vi "Checkers Main Menu.vi"() -> ()   [LabVIEW 2016]
uses:
  Game Info Global Variable.vi
panel:
  in  "SETTINGS":bool
  in  "HOW TO PLAY":bool
  in  "Comp Name:":string="Computer"
  in  "LOAD SAVED GAME":bool
  in  "Player 2 Name:":string="Player 2"
  in  "Player 1 Name:":string="Player 1"
  in  "Enum":T1(ring)
  in  "PLAY":bool
  in  "QUIT":bool
  in  "CREDITS":bool
  # "CHECKERS"
  # "A LabVIEW Project by Ritesh Misra and Daniel Sokolowski"
  # "Game Mode Select:"
  # "Player 1 Name:"
  # "Player 2 Name:"
  # "Computer \nOpponent Name:"
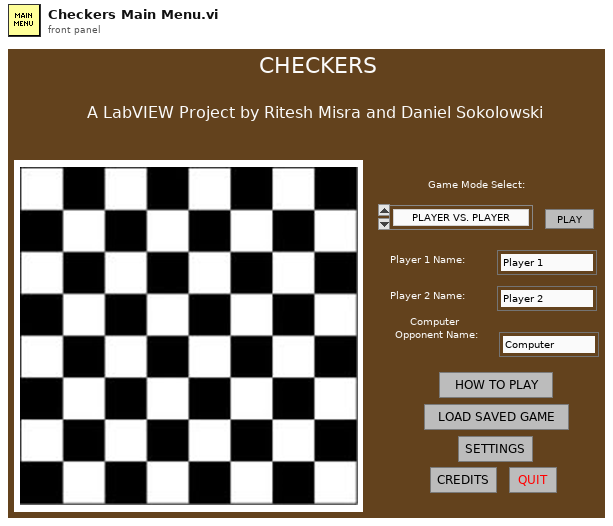
[diagram p1: front panel]
types:
  T1 = enum16{"PLAYER VS. PLAYER", "PLAYER VS. COMPUTER"}
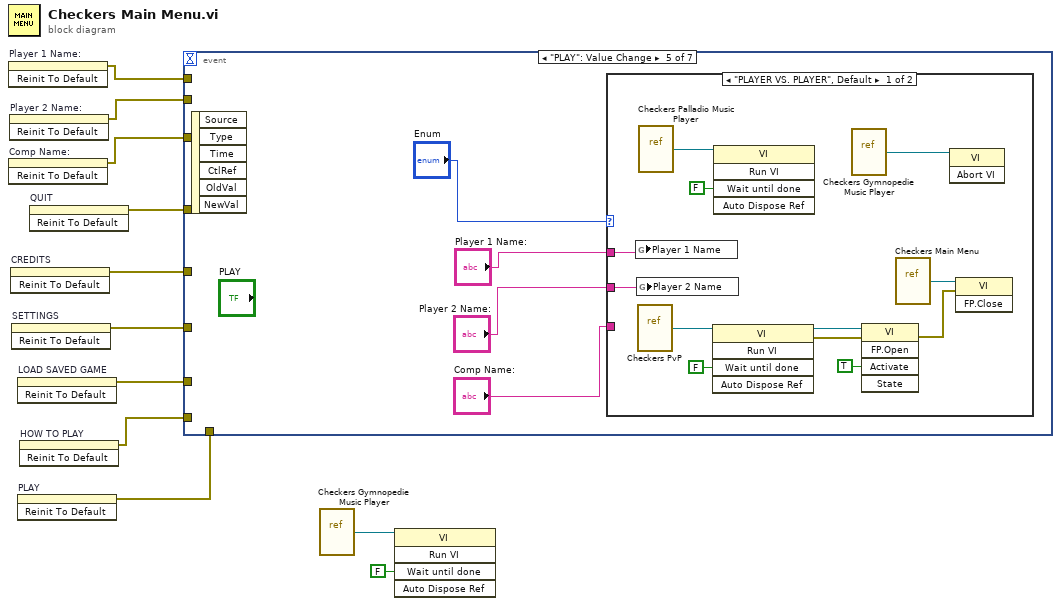
[diagram p0: block diagram]
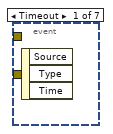
[diagram p2: hidden frame]
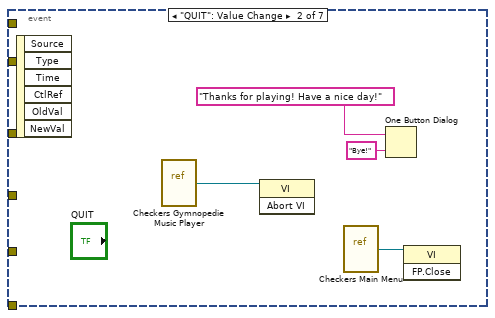
[diagram p3: hidden frame]
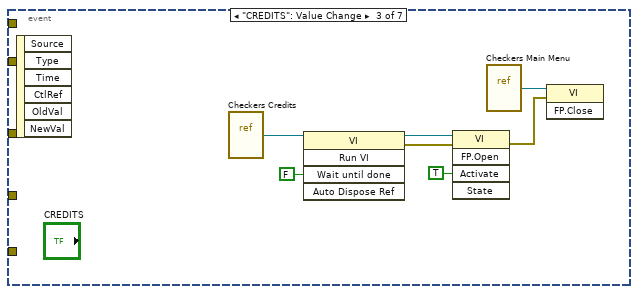
[diagram p4: hidden frame]
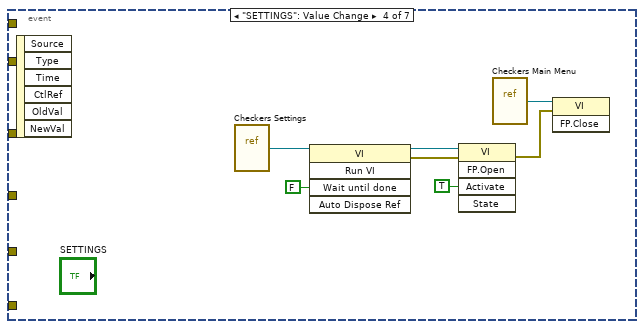
[diagram p5: hidden frame]
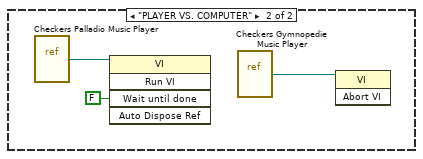
[diagram p6: hidden frame]
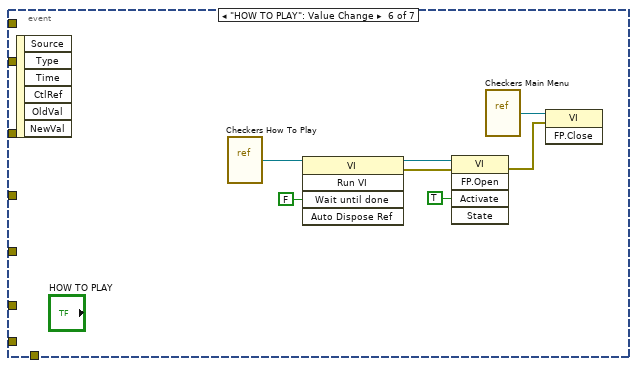
[diagram p7: hidden frame]
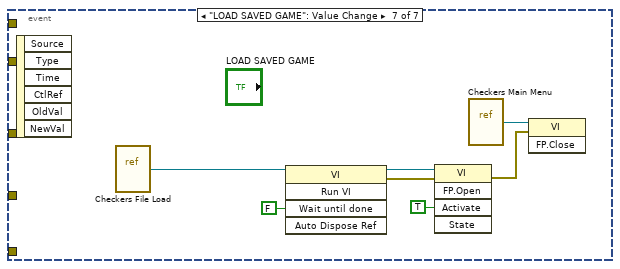
[diagram p8: hidden frame]
diagram:
  n1 = invoke on="Player 1 Name:" class="Str" method="Reinit To Default"() -> (error out=w5:errorcluster)  [unwired: 3 in, 2 out]
  n2 = invoke on="Comp Name:" class="Str" method="Reinit To Default"() -> (error out=w3:errorcluster)  [unwired: 3 in, 2 out]
  n3 = invoke on="Player 2 Name:" class="Str" method="Reinit To Default"() -> (error out=w4:errorcluster)  [unwired: 3 in, 2 out]
  n4 = invoke on="CREDITS" class="Bool" method="Reinit To Default"() -> (error out=w10:errorcluster)  [unwired: 3 in, 2 out]
  n5 = invoke on="SETTINGS" class="Bool" method="Reinit To Default"() -> (error out=w9:errorcluster)  [unwired: 3 in, 2 out]
  n6 = invoke on="LOAD SAVED GAME" class="Bool" method="Reinit To Default"() -> (error out=w8:errorcluster)  [unwired: 3 in, 2 out]
  n7 = invoke on="PLAY" class="Bool" method="Reinit To Default"() -> (error out=w6:errorcluster)  [unwired: 3 in, 2 out]
  n8 = invoke on="HOW TO PLAY" class="Bool" method="Reinit To Default"() -> (error out=w7:errorcluster)  [unwired: 3 in, 2 out]
  n9 = invoke on="QUIT" class="Bool" method="Reinit To Default"() -> (error out=w11:errorcluster)  [unwired: 3 in, 2 out]
  n10 = event shown="[4] \"PLAY\": Value Change" {
    selector: _ -> [_ _ _ _ _ _ _]
    dyn-events: _ -> [_ _ _ _ _ _ _]
    timeout: _ -> [_ _ _ _ _ _ _]
    tunnel: w11 -> [_ _ _ _ _ _ _]
    tunnel: w10 -> [_ _ _ _ _ _ _]
    tunnel: w9 -> [_ _ _ _ _ _ _]
    tunnel: w8 -> [_ _ _ _ _ _ _]
    tunnel: w7 -> [_ _ _ _ _ _ _]
    tunnel: w6 -> [_ _ _ _ _ _ _]
    tunnel: w5 -> [_ _ _ _ _ _ _]
    tunnel: w4 -> [_ _ _ _ _ _ _]
    tunnel: w3 -> [_ _ _ _ _ _ _]
    event Timeout {
      n11 = event-data() -> ()  [unwired: 1 in, 3 out]
    }
    event "QUIT": Value Change {
      n12 = event-data() -> ()  [unwired: 1 in, 6 out]
      n13 = vi-ref "Checkers Gymnopedie Music Player.vi"() -> (w12:refnum<vi>)
      n14 = invoke class="VI" method="Abort VI"(reference=w12) -> ()  [unwired: 2 in, 3 out]
      n15 = vi-ref "Checkers Main Menu.vi"() -> (w13:refnum<vi>)
      n16 = One Button Dialog(message="Thanks for playing! Have a nice day!", button name ("OK")="Bye!") -> ()  [unwired: 1 out]
      n17 = invoke class="VI" method="FP.Close"(reference=w13) -> ()  [unwired: 2 in, 3 out]
    }
    event "CREDITS": Value Change {
      n18 = event-data() -> ()  [unwired: 1 in, 6 out]
      n19 = vi-ref "Checkers Credits.vi"() -> (w22:refnum<vi>)
      n20 = invoke class="VI" method="Run VI"(reference=w22, "Wait until done"=FALSE ("Wait Until Done")) -> (reference out=w21:refnum<vi>, error out=w20:errorcluster)  [unwired: 3 in, 3 out]
      n21 = invoke class="VI" method="FP.Open"(reference=w21, error in=w20, "Activate"=TRUE ("Activate?")) -> (error out=w16:errorcluster)  [unwired: 2 in, 4 out]
      n22 = vi-ref "Checkers Main Menu.vi"() -> (w17:refnum<vi>)
      n23 = invoke class="VI" method="FP.Close"(reference=w17, error in=w16) -> ()  [unwired: 1 in, 3 out]
    }
    event "SETTINGS": Value Change {
      n24 = event-data() -> ()  [unwired: 1 in, 6 out]
      n25 = vi-ref "Checkers Settings.vi"() -> (w29:refnum<vi>)
      n26 = invoke class="VI" method="Run VI"(reference=w29, "Wait until done"=FALSE ("Wait Until Done")) -> (reference out=w28:refnum<vi>, error out=w27:errorcluster)  [unwired: 3 in, 3 out]
      n27 = invoke class="VI" method="FP.Open"(reference=w28, error in=w27, "Activate"=TRUE ("Activate?")) -> (error out=w23:errorcluster)  [unwired: 2 in, 4 out]
      n28 = vi-ref "Checkers Main Menu.vi"() -> (w24:refnum<vi>)
      n29 = invoke class="VI" method="FP.Close"(reference=w24, error in=w23) -> ()  [unwired: 1 in, 3 out]
    }
    event "PLAY": Value Change {
      n30 = event-data() -> ()  [unwired: 1 in, 6 out]
      n31 = case shown="\"PLAYER VS. PLAYER\", Default" "Enum" {
        tunnel: "Player 1 Name:" -> [w38 _]
        tunnel: "Player 2 Name:" -> [w37 _]
        tunnel: "Comp Name:" -> [_ _]
        frame "PLAYER VS. PLAYER", Default {
          n32 = global write "Game Info Global Variable.vi" "Player 1 Name"(w38) -> ()
          n33 = global write "Game Info Global Variable.vi" "Player 2 Name"(w37) -> ()
          n34 = vi-ref "Checkers PvP.vi"() -> (w45:refnum<vi>)
          n35 = vi-ref "Checkers Palladio Music Player.vi"() -> (w36:refnum<vi>)
          n36 = invoke class="VI" method="Run VI"(reference=w45, "Wait until done"=FALSE ("Wait Until Done")) -> (reference out=w44:refnum<vi>, error out=w43:errorcluster)  [unwired: 3 in, 3 out]
          n37 = invoke class="VI" method="Run VI"(reference=w36, "Wait until done"=FALSE ("Wait Until Done")) -> ()  [unwired: 3 in, 5 out]
          n38 = vi-ref "Checkers Gymnopedie Music Player.vi"() -> (w34:refnum<vi>)
          n39 = invoke class="VI" method="FP.Open"(reference=w44, error in=w43, "Activate"=TRUE ("Activate?")) -> (error out=w39:errorcluster)  [unwired: 2 in, 4 out]
          n40 = vi-ref "Checkers Main Menu.vi"() -> (w40:refnum<vi>)
          n41 = invoke class="VI" method="Abort VI"(reference=w34) -> ()  [unwired: 2 in, 3 out]
          n42 = invoke class="VI" method="FP.Close"(reference=w40, error in=w39) -> ()  [unwired: 1 in, 3 out]
        }
        frame "PLAYER VS. COMPUTER" {
          n43 = vi-ref "Checkers Palladio Music Player.vi"() -> (w48:refnum<vi>)
          n44 = invoke class="VI" method="Run VI"(reference=w48, "Wait until done"=FALSE ("Wait Until Done")) -> ()  [unwired: 3 in, 5 out]
          n45 = vi-ref "Checkers Gymnopedie Music Player.vi"() -> (w46:refnum<vi>)
          n46 = invoke class="VI" method="Abort VI"(reference=w46) -> ()  [unwired: 2 in, 3 out]
        }
      }
    }
    event "HOW TO PLAY": Value Change {
      n47 = event-data() -> ()  [unwired: 1 in, 6 out]
      n48 = vi-ref "Checkers How To Play.vi"() -> (w55:refnum<vi>)
      n49 = invoke class="VI" method="Run VI"(reference=w55, "Wait until done"=FALSE ("Wait Until Done")) -> (reference out=w54:refnum<vi>, error out=w53:errorcluster)  [unwired: 3 in, 3 out]
      n50 = invoke class="VI" method="FP.Open"(reference=w54, error in=w53, "Activate"=TRUE ("Activate?")) -> (error out=w49:errorcluster)  [unwired: 2 in, 4 out]
      n51 = vi-ref "Checkers Main Menu.vi"() -> (w50:refnum<vi>)
      n52 = invoke class="VI" method="FP.Close"(reference=w50, error in=w49) -> ()  [unwired: 1 in, 3 out]
    }
    event "LOAD SAVED GAME": Value Change {
      n53 = event-data() -> ()  [unwired: 1 in, 6 out]
      n54 = vi-ref "Checkers File Load.vi"() -> (w62:refnum<vi>)
      n55 = invoke class="VI" method="Run VI"(reference=w62, "Wait until done"=FALSE ("Wait Until Done")) -> (reference out=w61:refnum<vi>, error out=w60:errorcluster)  [unwired: 3 in, 3 out]
      n56 = invoke class="VI" method="FP.Open"(reference=w61, error in=w60, "Activate"=TRUE ("Activate?")) -> (error out=w56:errorcluster)  [unwired: 2 in, 4 out]
      n57 = vi-ref "Checkers Main Menu.vi"() -> (w57:refnum<vi>)
      n58 = invoke class="VI" method="FP.Close"(reference=w57, error in=w56) -> ()  [unwired: 1 in, 3 out]
    }
  }
  n59 = vi-ref "Checkers Gymnopedie Music Player.vi"() -> (w2:refnum<vi>)
  n60 = invoke class="VI" method="Run VI"(reference=w2, "Wait until done"=FALSE ("Wait Until Done")) -> ()  [unwired: 3 in, 5 out]
